vi "(SubVI) Marko-Sigga WLC fitting.vi"(4 "Force (pN)":dbl[](array[numeric]), 5 "Extension (nm)":dbl[](array[numeric]), 7 "initial parameters for marko":dbl[](array[numeric])=[40.0, 1800.0]) -> (0 "Extension to fit":dbl[](array[numeric]), 1 "r^2":dbl, 2 "best nonlinear fit for Force (pN)":dbl[](array[numeric]), 3 "best fit parameters\n(Lp,Lc)":dbl[](array[numeric]))   [LabVIEW 2014]
uses:
  <vilib>/gmath/NumericalOptimization/Nonlinear Curve Fit LM formula string.vi
  <vilib>/gmath/NI_Gmath.lvlib
panel:
  out "residue":dbl
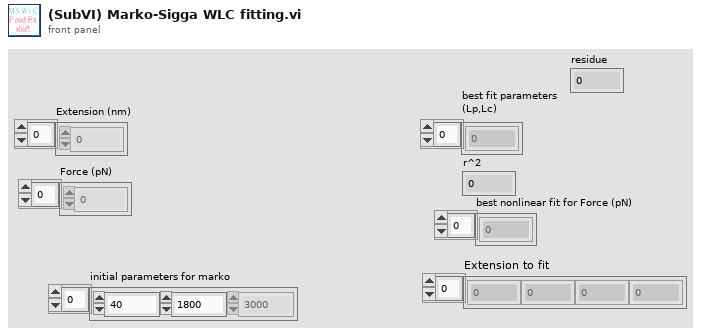
[diagram p1: front panel]
types:
  T1 = cluster{"model":string, "Parameters":string[], "x":string}
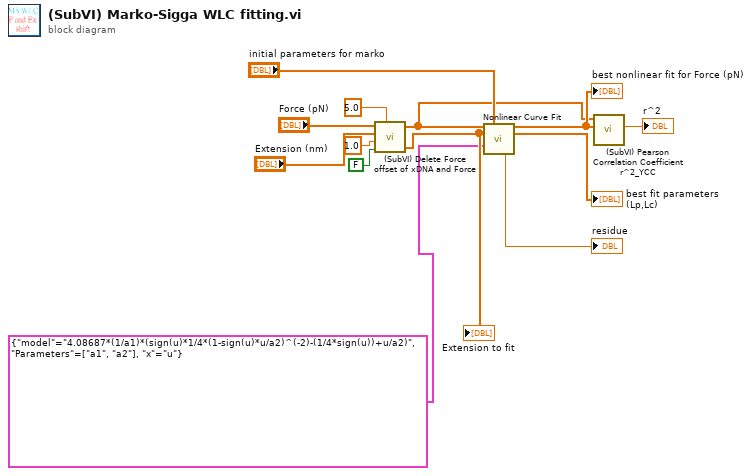
[diagram p0: block diagram]
diagram:
  n1 = call "(SubVI) Delete Force offset of xDNA and Force.vi"("Force"="Force (pN)", "Upper Force (pN)"=5.0, "xDNA"="Extension (nm)", "force constant"=1.0, "Set lower foce offset?"=FALSE) -> ("cut-full Force"=w3:dbl[], "cut-full xDNA"=w2:dbl[])  [unwired: 2 in]
  "Extension to fit" <- w2
  n2 = call-poly <vilib>:"Nonlinear Curve Fit.vi"("Y"=w3, "initial parameters"="initial parameters for marko", "X"=w2, "model description"=T1 {"model"="4.08687*(1/a1)*(sign(u)*1/4*(1-sign(u)*u/a2)^(-2)-(1/4*sign(u))+u/a2)", "Parameters"=["a1", "a2"], "x"="u"}) -> ("best nonlinear fit"=w10:dbl[], "best fit parameters"=→"best fit parameters\n(Lp,Lc)":dbl[], "residue"=→"residue":dbl)  [unwired: 3 in, 6 out]
  "best nonlinear fit for Force (pN)" <- w10
  n3 = call "(SubVI) Pearson Correlation Coefficient r^2_YCC.vi"("best fit Data"=w10, "Data"=w3) -> ("r^2"=→"r^2":dbl)  [unwired: 4 in, 1 out]
